vi "TellChild.vi"(6 "Error":errorcluster, 7 "Actor":refnum<class "Actor.lvclass">, 9 "Alias":string, 10 "MsgDVR":refnum<data-value>, 11 "Actor":T1) -> (3 "Actor":T1, 4 "Error":errorcluster, 5 "Actor":refnum<class "Actor.lvclass">)   [LabVIEW 2020, in "jettl.lvlib"]
uses:
  jettl.lvlib
  Msg/Msg.lvclass
  Metadata/Metadata.lvclass
  Actor/Actor.lvclass
  Origin.ctl
  Msg.ctl
  PostSetup.ctl
  PreSetup.ctl
  MsgNames.ctl
  Lifecycle.ctl
  ActorAttribs.ctl
  ChildActors.ctl
  Actor.ctl
  MsgAttribs.ctl
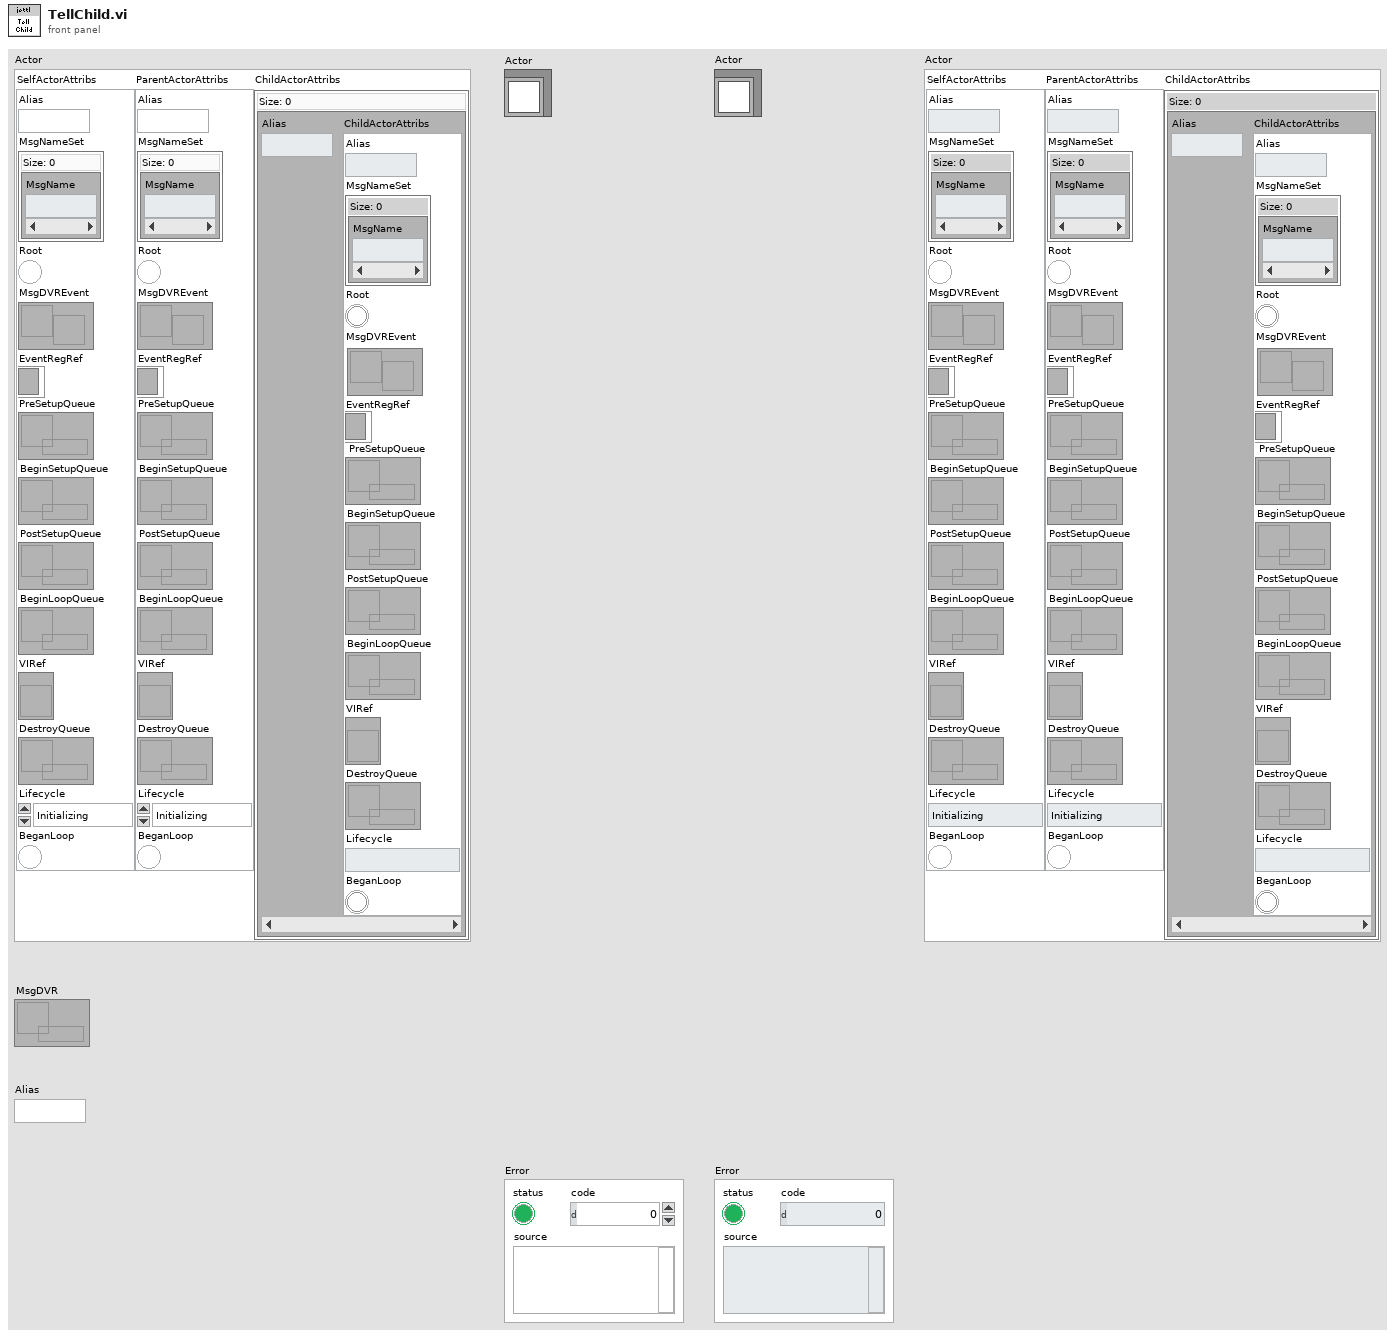
[diagram p1: front panel]
types:
  T1 = typedef "jettl.lvlib/Actor.ctl" = cluster{"SelfActorAttribs":T2, "ParentActorAttribs":T2, "ChildActorAttribs":T5}
  T2 = typedef "jettl.lvlib/ActorAttribs.ctl" = cluster{"Alias":string, "MsgNameSet":T3, "Root":bool, "MsgDVREvent":refnum<user-event>, "EventRegRef":refnum<event-registration>, "PreSetupQueue":refnum<queue>, "BeginSetupQueue":refnum<queue>, "PostSetupQueue":refnum<queue>, "BeginLoopQueue":refnum<queue>, "VIRef":refnum<vi>, "DestroyQueue":refnum<queue>, "Lifecycle":T4, "BeganLoop":bool}
  T3 = typedef "jettl.lvlib/MsgNames.ctl" = set{string}
  T4 = typedef "jettl.lvlib/Lifecycle.ctl" = enum16{"Initializing", "SettingUp", "Starting", "Running", "Stopping", "TearingDown", "Terminated"}
  T5 = typedef "jettl.lvlib/ChildActors.ctl" = map{string, T2}
  T6 = typedef "jettl.lvlib/Origin.ctl" = enum16{"Self", "Parent", "Child"}
  T7 = typedef "jettl.lvlib/MsgSet.ctl" = set{refnum<class "Message.lvclass">}
  T8 = typedef "jettl.lvlib/PreTell.ctl" = cluster{"MsgAttribsDVR":refnum<data-value>, "Msg":refnum<class "Msg.lvclass">}
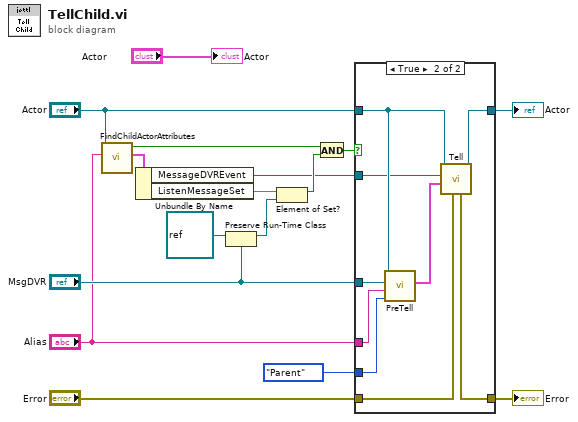
[diagram p0: block diagram]
diagram:
  n1 = call "FindChildActorAttributes.vi"("Alias"="Alias", "Actor"="Actor") -> ("ChildActorAttributes"=w8:T2, "Found"=w7:bool)  [unwired: 8 in]
  n2 = Unbundle By Name(w8) -> ("MessageDVREvent"=w4:refnum<user-event>, "ListenMessageSet"=w9:T7)
  n3 = Preserve Run-Time Class(object in=refnum<class> refnum, 2:"MsgDVR") -> (object out=w11:refnum<class "Msg.lvclass">)  [unwired: 1 in, 1 out]
  n4 = Element of Set?(10:w11, 11:w9) -> (3:w15:bool)
  n5 = And(x=w7, y=w15) -> (x .and. y?=w14:bool)
  n6 = case shown="True" w14 {
    tunnel: "Actor" -> [w18 w25]
    tunnel: [w18 w27] -> w16
    tunnel: "Alias" -> [_ w22]
    tunnel: "MsgDVR" -> [_ w26]
    tunnel: Origin."Parent" ("TellOrigin") -> [_ w23]
    tunnel: w4 -> [_ w24]
    tunnel: "Error" -> [w17 w20]
    tunnel: [w17 w19] -> w2
    frame False {
    }
    frame True {
      n7 = call "PreTell.vi"("Origin"=w23, "ListenerAlias"=w22, "MsgPreTell"=w26, "ActorDVR"=w25) -> ("MsgPreTell"=w21:T8)  [unwired: 6 in, 1 out]
      n8 = call "Tell.vi"("Error"=w20, "MsgPreTell"=w21, "MessageClusterDVREvent"=w24, "Actor"=w25) -> ("Actor"=w27:refnum<class "Actor.lvclass">, "Error"=w19:errorcluster)  [unwired: 6 in]
    }
  }
  "Actor" <- w16
  "Error" <- w2
  "Actor" <- "Actor"
